vi "获取本月一号日期.vi"() -> (3 "月一号":string)   [LabVIEW 2017]
panel:
  in  "日期格式":string="/"
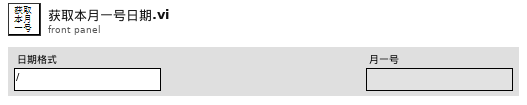
[diagram p1: front panel]
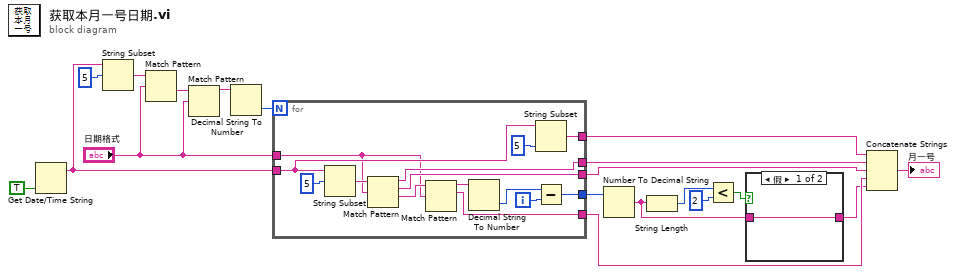
[diagram p0: block diagram]
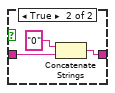
[diagram p2: hidden frame]
diagram:
  n1 = Get Date/Time String(want seconds? (F)=TRUE ("需要秒？(F)")) -> (date string=w7:string)  [unwired: 2 in, 1 out]
  n2 = String Subset(string=w7, offset (0)=5 ("偏移量(0)")) -> (substring=w10:string)  [unwired: 1 in]
  n3 = Match Pattern(string=w10, regular expression="日期格式") -> (after substring=w11:string)  [unwired: 1 in, 3 out]
  n4 = Match Pattern(string=w11, regular expression="日期格式") -> (before substring=w12:string)  [unwired: 1 in, 3 out]
  n5 = Decimal String To Number(string=w12) -> (number=w14:i32)  [unwired: 2 in, 1 out]
  n6 = for {
    N: w14 -> [_]
    tunnel: [w33] -> w16
    tunnel: [w32] -> w15
    tunnel: [w31] -> w18
    tunnel: [w22] -> w19
    tunnel: [w30] -> w17
    tunnel: w7 -> [w21]
    tunnel: "日期格式" -> [w20]
    i -> [w29]
    n7 = String Subset(string=w21, offset (0)=5 ("偏移量(0)")) -> (substring=w27:string)  [unwired: 1 in]
    n8 = Match Pattern(string=w27, regular expression=w20) -> (before substring=w31:string, match substring=w22:string, after substring=w25:string)  [unwired: 1 in, 1 out]
    n9 = Match Pattern(string=w25, regular expression=w20) -> (before substring=w24:string, match substring=w30:string)  [unwired: 1 in, 2 out]
    n10 = Decimal String To Number(string=w24) -> (number=w23:i32)  [unwired: 2 in, 1 out]
    n11 = String Subset(string=w21, length (rest)=5 ("偏移量(0)")) -> (substring=w32:string)  [unwired: 1 in]
    n12 = Subtract(x=w23, y=w29) -> (x-y=w33:i32)
  }
  n13 = Number To Decimal String(number=w16) -> (decimal integer string=w2:string)  [unwired: 1 in]
  n14 = String Length(string=w2) -> (length=w5:i32)
  n15 = Less?(x=w5, y=2) -> (x < y?=w3:bool)
  n16 = case shown="假" w3 {
    tunnel: w2 -> [w34 w37]
    tunnel: [w34 w35] -> w1
    frame False {
    }
    frame True {
      n17 = Concatenate Strings("0" ("字符串"), w37) -> (w35:string)
    }
  }
  n18 = Concatenate Strings(w15, w18, w19, w17, w1) -> (→"月一号":string)
